vi "상태머신_차선변경(11.25).vi"() -> ()   [LabVIEW 2018]
panel:
  in  "전방 장애물 발견!":bool
  in  "로깅 정지":bool
  out "코스판별":dbl
  out "E-Stop":bool
  in  "Logging On/Off":bool
  in  "Logging 저장위치":path
  out "상태결정":T1(ring)
  in  "설정 반지름":dbl
  out "주행완료":bool
  out "out":bool
  out "중간":bool
  out "in":bool
  out "직선":bool
  out "곡선":bool
  out "좌우 장애물":bool
  out "in 장애물":bool
  out "전방장애물":bool
  in  "in out 목표지정":bool
  in  "Gear":dbl
  in  "Brake":dbl
  in  "Speed":dbl
  in  "Steer":dbl
  out "GPS Speed":dbl
  out "GPS Steer":dbl
  # "<Lidar>"
  # "<Control>"
  # "<상태>"
  # "<GPS>"
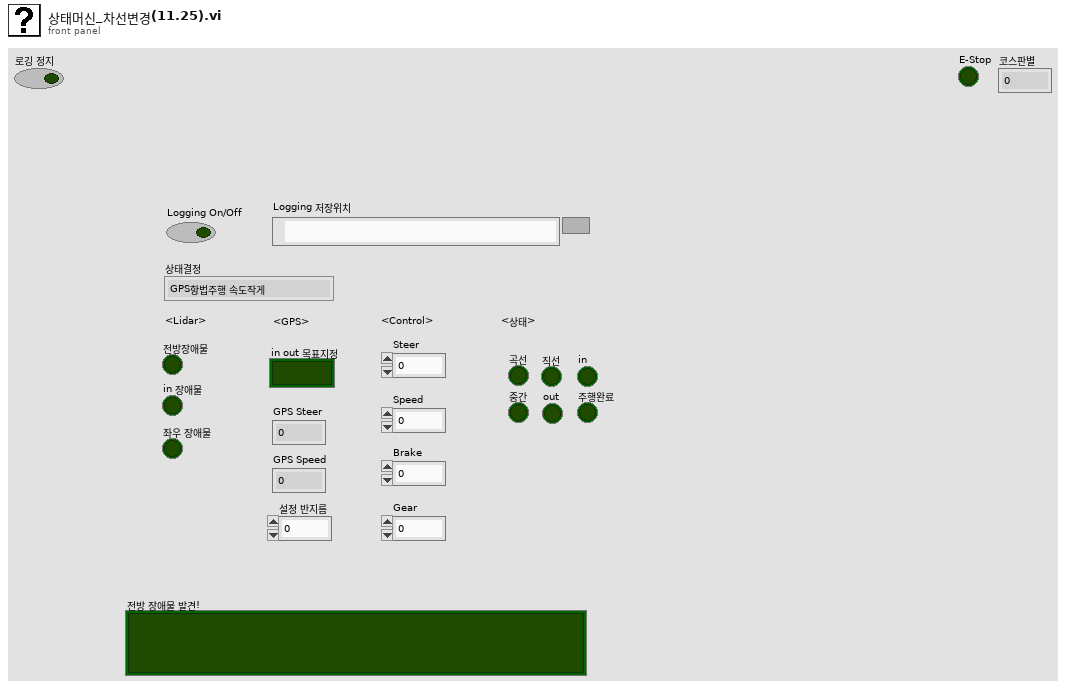
[diagram p1: front panel]
types:
  T1 = enum16{"GPS항법주행 속도작게", "out에서 in 차선변경", "in에서 out 차선변경", "멈춤", "GPS항법주행", "반지름축소"}
  T2 = cluster{dbl, dbl, "left(2) 2":bool, "go and left(1) 2":bool, "left(2) 3":bool, "left(2) 4":bool, "left(2) 5":bool, "left(2) 6":bool, dbl}
  T3 = cluster{"left(2)":bool, "left(2) 2":bool, "left(2) 3":bool}
  T4 = enum16{"GPS항법주행 속도작게", "out에서 in 차선변경", "in에서 out 차선변경", "멈춤", "GPS항법주행"}
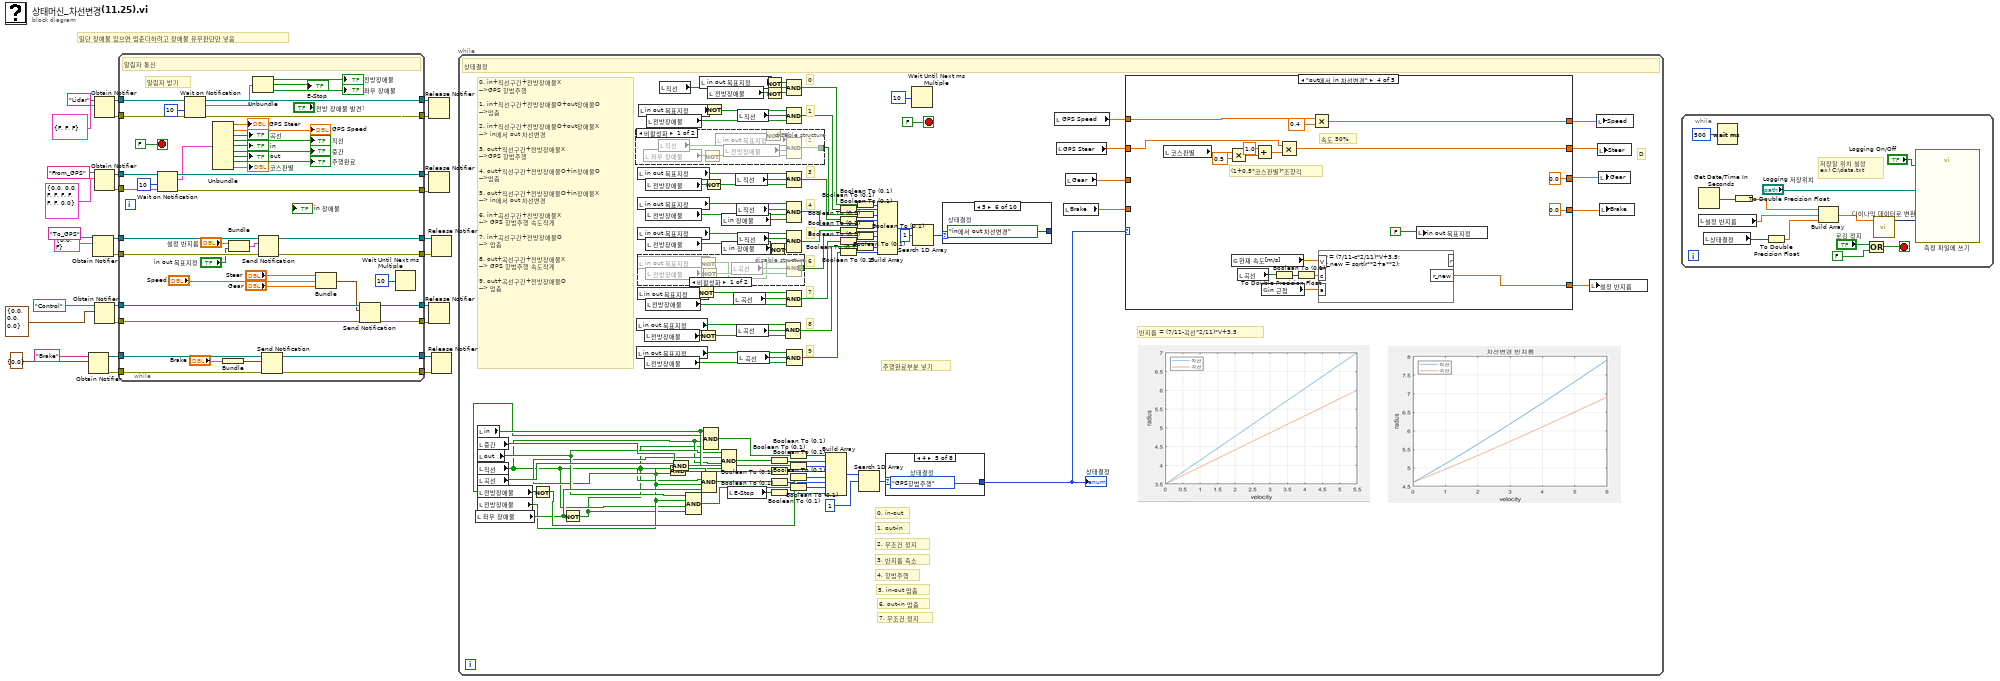
[diagram p0: block diagram]
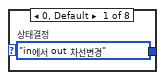
[diagram p2: hidden frame]
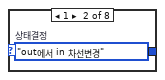
[diagram p3: hidden frame]
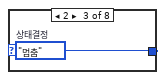
[diagram p4: hidden frame]
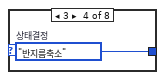
[diagram p5: hidden frame]
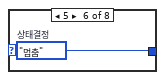
[diagram p6: hidden frame]
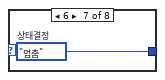
[diagram p7: hidden frame]
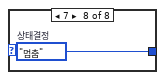
[diagram p8: hidden frame]
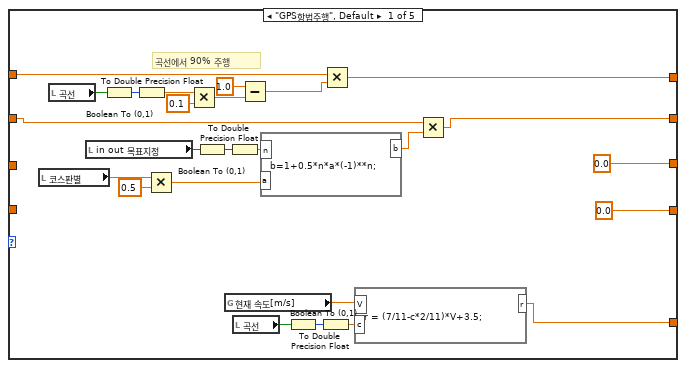
[diagram p9: hidden frame]
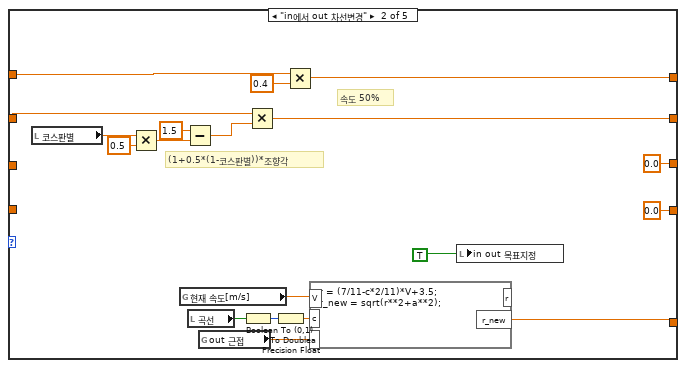
[diagram p10: hidden frame]
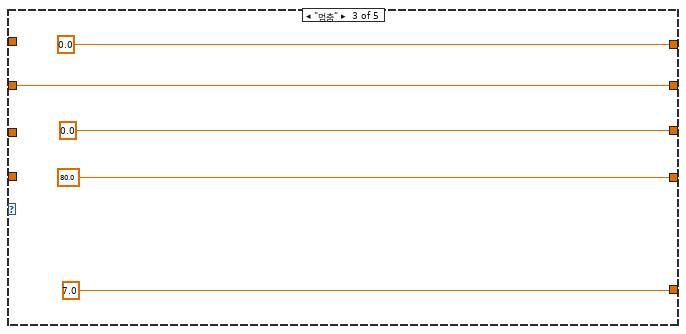
[diagram p11: hidden frame]
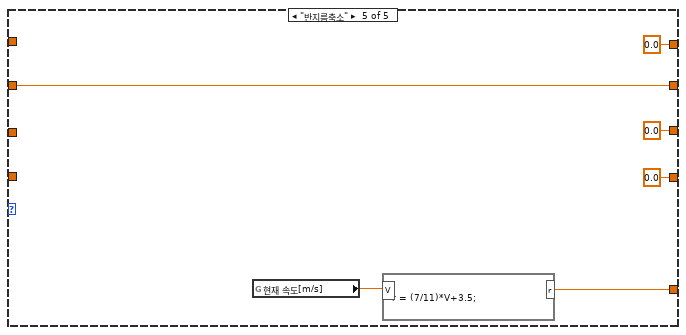
[diagram p12: hidden frame]
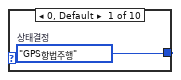
[diagram p15: hidden frame]
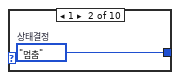
[diagram p16: hidden frame]
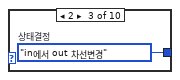
[diagram p17: hidden frame]
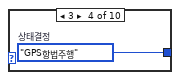
[diagram p18: hidden frame]
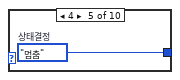
[diagram p19: hidden frame]
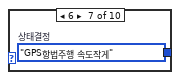
[diagram p20: hidden frame]
diagram:
  # "일단 장애물 있으면 멈춘다하려고 장애물 유무판단만 넣음"
  n1 = Obtain Notifier(name (unnamed)="Brake" ("이름(이름없음)"), notification data type=cluster{dbl} {0.0}) -> (notifier out=w4:refnum<notifier>, error out=w3:errorcluster)  [unwired: 2 in, 1 out]
  n2 = Obtain Notifier(name (unnamed)="To_GPS" ("이름(이름없음)"), notification data type=cluster{dbl, "left(2) 3":bool} {0.0, "left(2) 3"=FALSE}) -> (notifier out=w11:refnum<notifier>, error out=w10:errorcluster)  [unwired: 2 in, 1 out]
  n3 = Obtain Notifier(name (unnamed)="Lidar" ("이름(이름없음)"), notification data type=T3 {"left(2)"=FALSE, "left(2) 2"=FALSE, "left(2) 3"=FALSE}) -> (notifier out=w28:refnum<notifier>, error out=w26:errorcluster)  [unwired: 2 in, 1 out]
  n4 = Obtain Notifier(name (unnamed)="From_GPS" ("이름(이름없음)"), notification data type=T2 {0.0, 0.0, "left(2) 2"=FALSE, "go and left(1) 2"=FALSE, "left(2) 3"=FALSE, "left(2) 4"=FALSE, "left(2) 5"=FALSE, "left(2) 6"=FALSE, 0.0}) -> (notifier out=w24:refnum<notifier>, error out=w23:errorcluster)  [unwired: 2 in, 1 out]
  n5 = Obtain Notifier(name (unnamed)="Control" ("이름(이름없음)"), notification data type=cluster{dbl, dbl, dbl} {0.0, 0.0, 0.0}) -> (notifier out=w17:refnum<notifier>, error out=w18:errorcluster)  [unwired: 2 in, 1 out]
  n6 = while {
    tunnel: w28 -> [w77]
    tunnel: [w76] -> w27
    tunnel: w26 -> [w75]
    tunnel: [w74] -> w25
    tunnel: w24 -> [w73]
    tunnel: w23 -> [w72]
    tunnel: [w71] -> w22
    tunnel: [w70] -> w21
    tunnel: w17 -> [w63]
    tunnel: w18 -> [w64]
    tunnel: [w65] -> w19
    tunnel: [w66] -> w20
    tunnel: w11 -> [w46]
    tunnel: w10 -> [w47]
    tunnel: [w45] -> w9
    tunnel: [w44] -> w8
    tunnel: w4 -> [w35]
    tunnel: w3 -> [w32]
    tunnel: [w34] -> w2
    tunnel: [w33] -> w1
    stop <- FALSE stop-if-true
    # "알림자 받기"
    # "알림자 통신"
    n7 = Wait on Notification(notifier=w73, timeout in ms (-1)=10 ("타임아웃(ms) (-1)"), error in (no error)=w72) -> (notifier out=w70:refnum<notifier>, notification=w56:T2, error out=w71:errorcluster)  [unwired: 1 in, 1 out]
    n8 = Wait on Notification(notifier=w77, timeout in ms (-1)=10 ("타임아웃(ms) (-1)"), error in (no error)=w75) -> (notifier out=w76:refnum<notifier>, notification=w58:T3, error out=w74:errorcluster)  [unwired: 1 in, 1 out]
    n9 = Unbundle(w56) -> (→"GPS Steer":dbl, →"GPS Speed":dbl, "left(2) 2"=→"곡선":bool, "go and left(1) 2"=→"직선":bool, "left(2) 3"=→"in":bool, "left(2) 4"=→"중간":bool, "left(2) 5"=→"out":bool, "left(2) 6"=→"주행완료":bool, →"코스판별":dbl)
    n10 = Bundle("Brake"="Brake") -> (w36:cluster{"Brake":dbl})  [unwired: 1 in]
    n11 = Bundle("설정 반지름"="설정 반지름", "in out 목표지정"="in out 목표지정") -> (w41:cluster{"설정 반지름":dbl, "in out 목표지정":bool})  [unwired: 1 in]
    n12 = Unbundle(w58) -> ("left(2)"=→"전방장애물":bool, "left(2) 2"=→"E-Stop":bool, "left(2) 3"=→"좌우 장애물":bool)
    n13 = Send Notification(notification=w41, notifier=w46, error in (no error)=w47) -> (notifier out=w45:refnum<notifier>, error out=w44:errorcluster)
    n14 = Send Notification(notification=w36, notifier=w35, error in (no error)=w32) -> (notifier out=w34:refnum<notifier>, error out=w33:errorcluster)
    n15 = Bundle("Steer"="Steer", "Speed"="Speed", "Gear"="Gear") -> (w57:cluster{"Steer":dbl, "Speed":dbl, "Gear":dbl})  [unwired: 1 in]
    n16 = Send Notification(notification=w57, notifier=w63, error in (no error)=w64) -> (notifier out=w66:refnum<notifier>, error out=w65:errorcluster)
    n17 = Wait Until Next ms Multiple(millisecond multiple=u32 10 ("ms 배수")) -> ()  [unwired: 1 out]
  }
  n18 = Release Notifier(notifier=w27, error in (no error)=w25) -> ()  [unwired: 1 in, 3 out]
  n19 = Release Notifier(notifier=w21, error in (no error)=w22) -> ()  [unwired: 1 in, 3 out]
  n20 = Release Notifier(notifier=w20, error in (no error)=w19) -> ()  [unwired: 1 in, 3 out]
  n21 = Release Notifier(notifier=w9, error in (no error)=w8) -> ()  [unwired: 1 in, 3 out]
  n22 = Release Notifier(notifier=w2, error in (no error)=w1) -> ()  [unwired: 1 in, 3 out]
  n23 = while {
    stop <- FALSE stop-if-true
    # "반지름 = (7/11-곡선*2/11)*V+3.5"
    # "7. 무조건 정지"
    # "6. out-in 멈춤"
    # "5. in-out 멈춤"
    # "3. 반지름 축소"
    # "4. 항법주행"
    # "1. out-in"
    # "0. in-out"
    # "2. 무조건 정지"
    # "D"
    # "0. in+직선구간+전방장애물X\n-->GPS 항법주행\n\n1. in+직선구간+전방장애물O+out장애물O\n-->멈춤\n\n2. in+직선구간+전방장애물O+out장애물X\n--> in에서 out 차선변경\n\n3. out+직선구간+전방장애물X\n-->GPS 항법주행\n\n4. out+직선구간+전방장애물O+in장애물O\n-->멈춤\n\n5. out+직선구간+전방장애물O+in장애물X\n--> in에서 out 차선변경\n\n6. in+곡선구간+전방장애물X\n--> GPS 항법주행 속도작게\n\n7. in+곡선구간+전방장애물O\n--> 멈춤\n\n8. out+곡선구간+전방장애물X\n--> GPS 항법주행 속도작게\n\n9. out+곡선구간+전방장애물O\n--> 멈춤"
    # "주행완료부분 넣기"
    # "9"
    # "8"
    # "7"
    # "6"
    # "5"
    # "4"
    # "3"
    # "1"
    # "0"
    # "상태결정"
    n24 = local read "좌우 장애물"() -> (w89:bool)
    n25 = local read "in"() -> (w90:bool)
    n26 = local read "중간"() -> (w102:bool)
    n27 = local read "out"() -> (w86:bool)
    n28 = local read "직선"() -> (w84:bool)
    n29 = local read "곡선"() -> (w104:bool)
    n30 = local read "전방장애물"() -> (w103:bool)
    n31 = local read "전방장애물"() -> (w85:bool)
    n32 = Not(x=w103) -> (.not. x?=w92:bool)
    n33 = Not(x=w89) -> (.not. x?=w83:bool)
    n34 = disable-structure shown="비활성화" {
      disable-tunnel: [w264 _] -> w132
      frame Disabled {
        # "2"
        n35 = local read "좌우 장애물"() -> (w266:bool)
        n36 = local read "직선"() -> (w268:bool)
        n37 = Not(x=w266) -> (.not. x?=w265:bool)
        n38 = local read "in out 목표지정"() -> (w263:bool)
        n39 = local read "전방장애물"() -> (w267:bool)
        n40 = Not(x=w263) -> (.not. x?=w262:bool)
        n41 = Compound Arithmetic op=AND ("복합 연산")(w262, w268, w267, w265) -> (w264:bool)
      }
      frame Enabled {
      }
    }
    n42 = local read "in out 목표지정"() -> (w125:bool)
    n43 = local read "in out 목표지정"() -> (w126:bool)
    n44 = disable-structure shown="비활성화" {
      disable-tunnel: [w261 _] -> w160
      frame Disabled {
        n45 = local read "in out 목표지정"() -> (w257:bool)
        n46 = local read "전방장애물"() -> (w259:bool)
        n47 = Not(x=w257) -> (.not. x?=w256:bool)
        n48 = Not(x=w259) -> (.not. x?=w258:bool)
        n49 = local read "곡선"() -> (w260:bool)
        n50 = Compound Arithmetic op=AND ("복합 연산")(w256, w260, w258) -> (w261:bool)
      }
      frame Enabled {
      }
    }
    n51 = local read "in out 목표지정"() -> (w117:bool)
    n52 = local read "in out 목표지정"() -> (w122:bool)
    n53 = local read "in out 목표지정"() -> (w123:bool)
    n54 = local read "in out 목표지정"() -> (w124:bool)
    n55 = local read "in out 목표지정"() -> (w119:bool)
    n56 = local read "전방장애물"() -> (w128:bool)
    n57 = local read "전방장애물"() -> (w143:bool)
    n58 = local read "전방장애물"() -> (w145:bool)
    n59 = local read "전방장애물"() -> (w134:bool)
    n60 = local read "전방장애물"() -> (w155:bool)
    n61 = local read "전방장애물"() -> (w158:bool)
    n62 = local read "전방장애물"() -> (w159:bool)
    n63 = local read "직선"() -> (w164:bool)
    n64 = And(x=w102, y=w85) -> (x .and. y?=w93:bool)
    n65 = And(x=w104, y=w85) -> (x .and. y?=w96:bool)
    n66 = Compound Arithmetic op=AND ("복합 연산")(w86, w85, w84, w83) -> (w82:bool)
    n67 = Not(x=w117) -> (.not. x?=w116:bool)
    n68 = Not(x=w128) -> (.not. x?=w127:bool)
    n69 = local read "in out 목표지정"() -> (w121:bool)
    n70 = Compound Arithmetic op=AND ("복합 연산")(w90, w84, w85, w89) -> (w88:bool)
    n71 = Not(x=w134) -> (.not. x?=w133:bool)
    n72 = Compound Arithmetic op=AND ("복합 연산")(w90, w85, w84, w83) -> (w100:bool)
    n73 = Not(x=w119) -> (.not. x?=w118:bool)
    n74 = local read "전방장애물"() -> (w135:bool)
    n75 = local read "in 장애물"() -> (w156:bool)
    n76 = Compound Arithmetic op=AND ("복합 연산")(w86, w85, w84, w83) -> (w97:bool)
    n77 = local read "in 장애물"() -> (w131:bool)
    n78 = local read "E-Stop"() -> (w79:bool)
    n79 = local read "곡선"() -> (w146:bool)
    n80 = local read "직선"() -> (w153:bool)
    n81 = local read "직선"() -> (w154:bool)
    n82 = local read "곡선"() -> (w140:bool)
    n83 = local read "직선"() -> (w162:bool)
    n84 = local read "직선"() -> (w157:bool)
    n85 = local read "곡선"() -> (w141:bool)
    n86 = Not(x=w121) -> (.not. x?=w120:bool)
    n87 = Not(x=w135) -> (.not. x?=w136:bool)
    n88 = Not(x=w131) -> (.not. x?=w130:bool)
    n89 = Boolean To (0,1)(Boolean=w97) -> (0, 1=w98:i16)
    n90 = Boolean To (0,1)(Boolean=w93) -> (0, 1=w94:i16)
    n91 = Boolean To (0,1)(Boolean=w88) -> (0, 1=w87:i16)
    n92 = Boolean To (0,1)(Boolean=w79) -> (0, 1=w78:i16)
    n93 = Compound Arithmetic op=AND ("복합 연산")(w125, w140, w127) -> (w139:bool)
    n94 = Compound Arithmetic op=AND ("복합 연산")(w120, w164, w136) -> (w163:bool)
    n95 = Compound Arithmetic op=AND ("복합 연산")(w118, w162, w159) -> (w161:bool)
    n96 = Compound Arithmetic op=AND ("복합 연산")(w122, w153, w133) -> (w152:bool)
    n97 = Compound Arithmetic op=AND ("복합 연산")(w123, w154, w155, w156) -> (w151:bool)
    n98 = Compound Arithmetic op=AND ("복합 연산")(w124, w157, w158, w130) -> (w149:bool)
    n99 = Compound Arithmetic op=AND ("복합 연산")(w116, w146, w145) -> (w129:bool)
    n100 = Compound Arithmetic op=AND ("복합 연산")(w126, w141, w143) -> (w142:bool)
    n101 = Boolean To (0,1)(Boolean=w100) -> (0, 1=w99:i16)
    n102 = Boolean To (0,1)(Boolean=w96) -> (0, 1=w95:i16)
    n103 = Boolean To (0,1)(Boolean=w92) -> (0, 1=w91:i16)
    n104 = Boolean To (0,1)(Boolean=w82) -> (0, 1=w81:i16)
    n105 = Build Array(w99, w98, w95, w94, w91, w87, w81, w78) -> (w107:i16[])
    n106 = Boolean To (0,1)(Boolean=w161) -> (0, 1=w169:i16)
    n107 = Boolean To (0,1)(Boolean=w152) -> (0, 1=w166:i16)
    n108 = Boolean To (0,1)(Boolean=w149) -> (0, 1=w148:i16)
    n109 = Boolean To (0,1)(Boolean=w129) -> (0, 1=w144:i16)
    n110 = Boolean To (0,1)(Boolean=w142) -> (0, 1=w137:i16)
    n111 = Boolean To (0,1)(Boolean=w163) -> (0, 1=w173:i16)
    n112 = Boolean To (0,1)(Boolean=w132) -> (0, 1=w167:i16)
    n113 = Boolean To (0,1)(Boolean=w151) -> (0, 1=w150:i16)
    n114 = Boolean To (0,1)(Boolean=w160) -> (0, 1=w147:i16)
    n115 = Boolean To (0,1)(Boolean=w139) -> (0, 1=w138:i16)
    n116 = Search 1D Array(1D array=w107, element=i16 1 ("원소")) -> (index of element=w106:i32)  [unwired: 1 in]
    n117 = Build Array(w173, w169, w167, w166, w150, w148, w147, w144, w138, w137) -> (w172:i16[])
    n118 = case shown="4" w106 {
      tunnel: [w174 w175 w176 w177 w178 w179 w180 w181] -> w80
      frame 0, Default {
        w174 = T1."in에서 out 차선변경"  # 상태결정
      }
      frame 1 {
        w175 = T1."out에서 in 차선변경"  # 상태결정
      }
      frame 2 {
        w176 = T1."멈춤"  # 상태결정
      }
      frame 3 {
        w177 = T1."반지름축소"  # 상태결정
      }
      frame 4 {
        w178 = T1."GPS항법주행"  # 상태결정
      }
      frame 5 {
        w179 = T1."멈춤"  # 상태결정
      }
      frame 6 {
        w180 = T1."멈춤"  # 상태결정
      }
      frame 7 {
        w181 = T1."멈춤"  # 상태결정
      }
    }
    "상태결정" <- w80
    n119 = Wait Until Next ms Multiple(millisecond multiple=u32 10 ("ms 배수")) -> ()  [unwired: 1 out]
    n120 = Search 1D Array(1D array=w172, element=i16 1 ("원소")) -> (index of element=w165:i32)  [unwired: 1 in]
    n121 = case shown="5" w165 {
      tunnel: [w269 w270 w271 w272 w273 w274 w275 w276 w277 w278] -> _
      frame 0, Default {
        w269 = T4."GPS항법주행"  # 상태결정
      }
      frame 1 {
        w270 = T4."멈춤"  # 상태결정
      }
      frame 2 {
        w271 = T4."in에서 out 차선변경"  # 상태결정
      }
      frame 3 {
        w272 = T4."GPS항법주행"  # 상태결정
      }
      frame 4 {
        w273 = T4."멈춤"  # 상태결정
      }
      frame 5 {
        w274 = T4."in에서 out 차선변경"  # 상태결정
      }
      frame 6 {
        w275 = T4."GPS항법주행 속도작게"  # 상태결정
      }
      frame 7 {
        w276 = T4."멈춤"  # 상태결정
      }
      frame 8 {
        w277 = T4."GPS항법주행 속도작게"  # 상태결정
      }
      frame 9 {
        w278 = T4."멈춤"  # 상태결정
      }
    }
    n122 = local read "GPS Speed"() -> (w108:dbl)
    n123 = local read "GPS Steer"() -> (w110:dbl)
    n124 = local read "Brake"() -> (w115:dbl)
    n125 = local read "Gear"() -> (w114:dbl)
    n126 = case shown="\"out에서 in 차선변경\"" w80 {
      tunnel: w108 -> [w196 w214 _ w239 _]
      tunnel: [w198 w215 0.0 ("Speed") w238 0.0 ("Speed")] -> w109
      tunnel: w110 -> [w188 w216 w229 w241 w255]
      tunnel: [w187 w222 w229 w240 w255] -> w111
      tunnel: [0.0 ("Gear") 0.0 ("Gear") 0.0 ("Speed") 0.0 ("Gear") 0.0 ("Gear")] -> w112
      tunnel: [0.0 ("Gear") 0.0 ("Brake") 80.0 ("Speed") 0.0 ("Brake") 0.0 ("Brake")] -> w113
      tunnel: w114 -> [_ _ _ _ _]
      tunnel: w115 -> [_ _ _ _ _]
      tunnel: [w182 w208 7.0 ("Speed") w232 w250] -> w105
      frame "GPS항법주행", Default {
        # "곡선에서 90% 주행"
        n127 = local read "코스판별"() -> (w195:dbl)
        n128 = local read "곡선"() -> (w204:bool)
        n129 = local read "in out 목표지정"() -> (w192:bool)
        n130 = Boolean To (0,1)(Boolean=w204) -> (0, 1=w203:i16)
        n131 = To Double Precision Float(number=w203) -> (double precision float=w202:dbl)
        n132 = Multiply(x=w195, y=0.5) -> (x*y=w190:dbl)
        n133 = Multiply(x=w202, y=0.1) -> (x*y=w200:dbl)
        n134 = Boolean To (0,1)(Boolean=w192) -> (0, 1=w193:i16)
        n135 = global read "글로벌 (11.25).vi" "현재 속도[m/s]"() -> (w184:dbl)
        n136 = To Double Precision Float(number=w193) -> (double precision float=w191:dbl)
        n137 = local read "곡선"() -> (w185:bool)
        n138 = Subtract(x=1.0, y=w200) -> (x-y=w197:dbl)
        n139 = formula code="b=1+0.5*n*a*(-1)**n;"("n"=w191, "a"=w190) -> ("b"=w189:dbl)
        n140 = Boolean To (0,1)(Boolean=w185) -> (0, 1=w186:i16)
        n141 = To Double Precision Float(number=w186) -> (double precision float=w183:dbl)
        n142 = Multiply(x=w196, y=w197) -> (x*y=w198:dbl)
        n143 = formula code="r = (7/11-c*2/11)*V+3.5;"("V"=w184, "c"=w183) -> ("r"=w182:dbl)
        n144 = Multiply(x=w188, y=w189) -> (x*y=w187:dbl)
      }
      frame "in에서 out 차선변경" {
        # "속도 50%"
        # "(1+0.5*(1-코스판별))*조향각"
        n145 = local read "코스판별"() -> (w220:dbl)
        n146 = Multiply(x=w220, y=0.5) -> (x*y=w218:dbl)
        n147 = global read "글로벌 (11.25).vi" "현재 속도[m/s]"() -> (w210:dbl)
        n148 = Subtract(x=1.5, y=w218) -> (x-y=w217:dbl)
        n149 = local read "곡선"() -> (w211:bool)
        n150 = global read "글로벌 (11.25).vi" "out 근접"() -> (w207:dbl)
        n151 = Boolean To (0,1)(Boolean=w211) -> (0, 1=w212:i16)
        n152 = Multiply(x=w216, y=w217) -> (x*y=w222:dbl)
        n153 = To Double Precision Float(number=w212) -> (double precision float=w209:dbl)
        n154 = Multiply(x=w214, y=0.4) -> (x*y=w215:dbl)
        n155 = formula code="r = (7/11-c*2/11)*V+3.5;\nr_new = sqrt(r**2+a**2);"("V"=w210, "c"=w209, "a"=w207) -> ("r_new"=w208:dbl)  [unwired: 1 out]
        n156 = local write "in out 목표지정"(TRUE ("in out 상태")) -> ()
      }
      frame "멈춤" {
      }
      frame "out에서 in 차선변경" {
        # "속도 50%"
        # "(1+0.5*코스판별)*조향각"
        n157 = local read "코스판별"() -> (w245:dbl)
        n158 = Multiply(x=w245, y=0.5) -> (x*y=w244:dbl)
        n159 = global read "글로벌 (11.25).vi" "현재 속도[m/s]"() -> (w234:dbl)
        n160 = local read "곡선"() -> (w235:bool)
        n161 = Add(x=1.0, y=w244) -> (x+y=w242:dbl)
        n162 = global read "글로벌 (11.25).vi" "in 근접"() -> (w231:dbl)
        n163 = Boolean To (0,1)(Boolean=w235) -> (0, 1=w236:i16)
        n164 = Multiply(x=w241, y=w242) -> (x*y=w240:dbl)
        n165 = To Double Precision Float(number=w236) -> (double precision float=w233:dbl)
        n166 = Multiply(x=w239, y=0.4) -> (x*y=w238:dbl)
        n167 = formula code="r = (7/11-c*2/11)*V+3.5;\nr_new = sqrt(r**2+a**2);"("V"=w234, "c"=w233, "a"=w231) -> ("r_new"=w232:dbl)  [unwired: 1 out]
        n168 = local write "in out 목표지정"(FALSE ("in out 상태")) -> ()
      }
      frame "반지름축소" {
        n169 = global read "글로벌 (11.25).vi" "현재 속도[m/s]"() -> (w251:dbl)
        n170 = formula code="r = (7/11)*V+3.5;"("V"=w251) -> ("r"=w250:dbl)
      }
    }
    n171 = local write "설정 반지름"(w105) -> ()
    n172 = local write "Speed"(w109) -> ()
    n173 = local write "Steer"(w111) -> ()
    n174 = local write "Gear"(w112) -> ()
    n175 = local write "Brake"(w113) -> ()
  }
  n176 = while {
    stop <- w281 stop-if-true
    # "저장할 위치 설정\nex) C:\\data.txt"
    n177 = Get Date/Time In Seconds() -> (seconds since 1Jan1904=w286:timestamp)
    n178 = local read "설정 반지름"() -> (w284:dbl)
    n179 = local read "상태결정"() -> (w283:T1)
    n180 = Wait (ms)(milliseconds to wait=u32 500 ("대기 시간 (ms)")) -> ()  [unwired: 1 out]
    n181 = To Double Precision Float(number=w286) -> (double precision float=w285:dbl)
    n182 = To Double Precision Float(number=w283) -> (double precision float=w282:dbl)
    n183 = Build Array(w285, w284, w282) -> (w287:dbl[])
    n184 = Or(x="로깅 정지", y=FALSE) -> (x .or. y?=w281:bool)
    n185 = call "다이나믹 데이터로 변환"("Array"=w287) -> ("Dynamic Data Type"=w290:dynamicdata)  [unwired: 3 in]
    n186 = call "측정 파일에 쓰기"("Signals"=w290, "Enable"="Logging On/Off", "Filename"="Logging 저장위치") -> ()  [unwired: 14 in, 3 out]
  }
